vi "Start Automatic Execution.vi"(8 "error in (no error)":errorcluster, 10 "Measuring Limb":string, 11 "Queue in":refnum<queue>) -> (0 "error out":errorcluster)   [LabVIEW 2013, in "main.lvlib"]
uses:
  main.lvlib
  Controls/Enum Variables.ctl
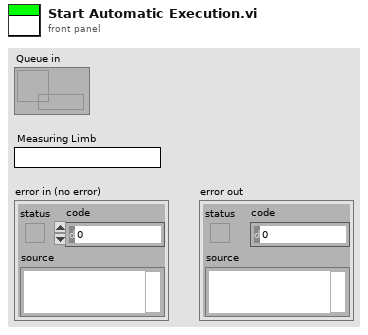
[diagram p1: front panel]
types:
  T1 = typedef "main.lvlib/Enum Variables.ctl" = enum16{"SetAcqFilter", "GetAcqFilter", "Set Filter", "Get Filter", "Set Height", "Get Height", "Set Recorded Height", "Get Recorded Height", "Set Blue Pressure", "Get Blue Pressure", "Set Red Pressure", "Get Red Pressure", "Init", "Reset Pressure", "Set Red Cursors", "Get Red Cursors", "Set Blue Cursors", "Get Blue Cursors", "Set Language", "Get Language", "Set Active Graphs", "Get ActiveGraphs", "Set Method", "Get Method", "Set Encryption", "Get Encryption", "Set ExcelVersion", "Get ExcelVersion", "Set DICOM Avail", "Get DICOM Avail", "Set DICOM Encode", "Get DICOM Encode", "Set JournalExport", "Get JournalExport", "Set Sequence", "Get Sequence", "Set DAQ Connected", "Get DAQ Connected", "Set Current Graph", "Get Current Graph", "Set General Settings", "Get Hyphenation", "Set Arm Calc Method", "Get Arm Calc Method", "Set Dicom Tags", "Get Dicom Tags", "Set BT Serial", "Get BT Serial", "Set BT Accepted Serials", "Get BT Accepted Serials", "Get BT License", "Set BT License"}
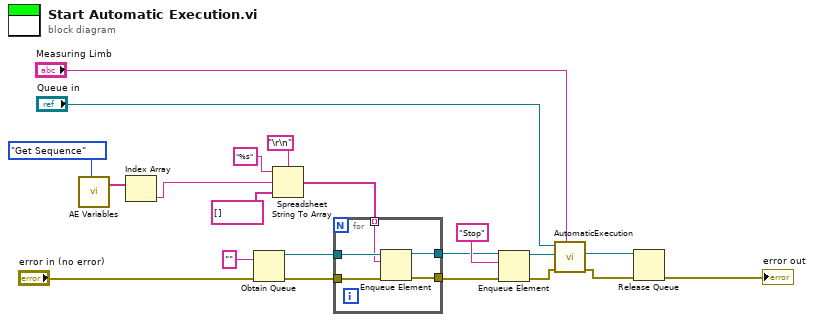
[diagram p0: block diagram]
diagram:
  n1 = call "AE Variables.vi"("Action"=Enum_Variables."Get Sequence") -> ("stringArray"=w20:string[])  [unwired: 11 in, 7 out]
  n2 = Index Array(array=w20) -> (element=w21:string)  [unwired: 1 in]
  n3 = Obtain Queue(element data type="", error in (no error)="error in (no error)") -> (queue out=w4:refnum<queue>, error out=w6:errorcluster)  [unwired: 3 in, 1 out]
  n4 = Spreadsheet String To Array(delimiter (Tab)="\r\n", format string="%s", spreadsheet string=w21, array type (2D Dbl)=string[] []) -> (array=w5:string[])
  n5 = for {
    tunnel: w4 -> [w26]
    tunnel: w5 -> [w25] mode=indexing
    tunnel: w6 -> [w24]
    tunnel: [w23] -> w15
    tunnel: [w22] -> w14
    n6 = Enqueue Element(queue=w26, element=w25, error in (no error)=w24) -> (queue out=w22:refnum<queue>, error out=w23:errorcluster)  [unwired: 1 in, 1 out]
  }
  n7 = Enqueue Element(queue=w14, element="Stop", error in (no error)=w15) -> (queue out=w16:refnum<queue>, error out=w17:errorcluster)  [unwired: 1 in, 1 out]
  n8 = call "AutomaticExecution.vi"("Measuring Limb"="Measuring Limb", "error in (no error)"=w17, "Automatic Queue"=w16, "Control.Queue"="Queue in") -> ("error out"=w12:errorcluster, "Automatic Queue out"=w11:refnum<queue>)  [unwired: 6 in]
  n9 = Release Queue(queue=w11, error in (no error)=w12) -> (error out=→"error out":errorcluster)  [unwired: 1 in, 2 out]
